vi "Start (Memory).vi"(7 "VolatusConfig":refnum<class "VolatusConfig.lvclass">, 8 "error in (no error)":errorcluster, 10 "Node Name":string) -> (0 "error out":errorcluster, 2 "MessageQ":refnum<class "MessageQ.lvclass">)   [LabVIEW 2020, in "Volatus.lvlib" / "Volatus Core.lvclass"]
uses:
  Volatus Core.lvclass
  Volatus Core.lvclass/Volatus Core.ctl
  Module/Module.lvclass
  VolatusAPI/VolatusAPI.lvclass
  VolatusConfig/VolatusConfig/VolatusConfig.lvclass
  Config Type.ctl
  VolatusConfig/Node/Node.lvclass
  C:/dev/lv20CE/relink/lv-volatus/Volatus/Module/Module.lvclass
  C:/dev/lv20CE/relink/lv-volatus/Volatus/Volatus Core/Volatus Core.lvclass
  C:/dev/lv20CE/relink/lv-volatus/VolatusConfig/VolatusConfigElement/VolatusConfigElement.lvclass
  C:/dev/lv20CE/relink/lv-volatus/VolatusConfig/Node/Node.lvclass
  MessageQ/MessageQ.lvclass
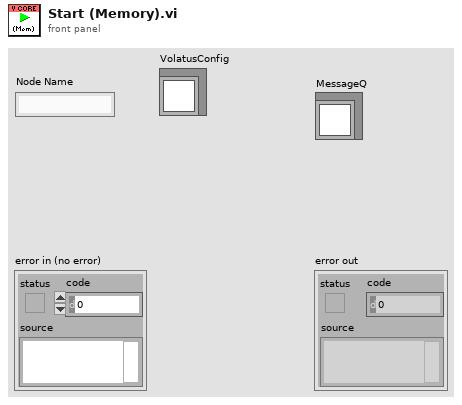
[diagram p1: front panel]
types:
  T1 = typedef "Volatus.lvlib/Volatus Core.lvclass/Config Type.ctl" = enum16{"App INI", "Memory"}
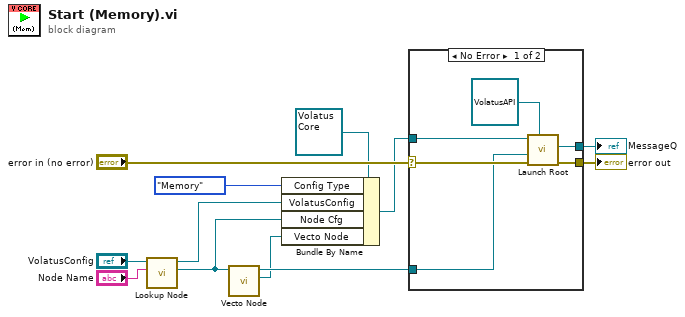
[diagram p0: block diagram]
diagram:
  n1 = call "Lookup Node.vi"("Node Name"="Node Name", "VolatusConfig in"="VolatusConfig") -> ("Node"=w3:refnum<class "Node.lvclass">, "VolatusConfig out"=w4:refnum<class "VolatusConfig.lvclass">)  [unwired: 7 in, 1 out]
  n2 = call "Vecto Node.vi"("Node in"=w3) -> ("Vecto Node"=w1:refnum<class "Node Config.lvclass">, "Node out"=w2:refnum<class "Node.lvclass">)  [unwired: 8 in, 1 out]
  n3 = Bundle By Name(cluster=refnum<class "Volatus Core.lvclass"> refnum ("Volatus Core in"), "Config Type"=Config_Type."Memory", "VolatusConfig"=w4, "Node Cfg"=w3, "Vecto Node"=w1) -> (w6:refnum<class "Volatus Core.lvclass">)
  n4 = case shown="No Error" "error in (no error)" {
    selector: "error in (no error)" -> [w18 w19]
    tunnel: [w17 w19] -> w11
    tunnel: [w16 _] -> w12
    tunnel: w6 -> [w15 _]
    tunnel: w2 -> [w13 _]
    frame No Error {
      n5 = call "Launch Root.vi"("VolatusAPI"=refnum<class "VolatusAPI.lvclass"> refnum, "error in (no error)"=w18, "Config Element"=w13, "Module in"=w15) -> ("error out"=w17:errorcluster, "MessageQ"=w16:refnum<class "MessageQ.lvclass">)  [unwired: 6 in]
    }
    frame Error {
    }
  }
  "error out" <- w11
  "MessageQ" <- w12
